vi "Page_Drivers_Write.vi"(6 "ctlReferences":T1, 8 "error in (no error)":errorcluster, 11 "IB_MSI in":refnum<class "IB_MSI.lvclass">) -> (0 "error out":errorcluster, 3 "IB_MSI out":refnum<class "IB_MSI.lvclass">)   [LabVIEW 2020, in "IB_MSI.lvclass"]
uses:
  <vilib>/AppBuilder/IB_Classes/MSI/IB_MSI.lvclass
  <vilib>/AppBuilder/IB_Classes/MSI/IB_MSI.lvclass/IB_MSI.ctl
  <resource>/Framework/Providers/Builds/Installer/Pages/controls/IB_UI_Page_Drivers_References.ctl
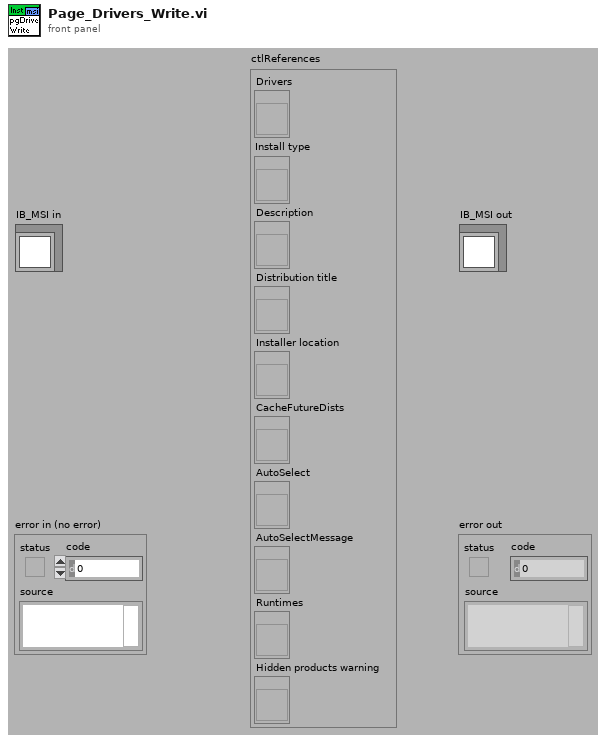
[diagram p1: front panel]
types:
  T1 = typedef "IB_UI_Page_Drivers_References.ctl" = cluster{"Drivers":refnum<vi>, "Install type":refnum<vi>, "Description":refnum<vi>, "Distribution title":refnum<vi>, "Installer location":refnum<vi>, "CacheFutureDists":refnum<vi>, "AutoSelect":refnum<vi>, "AutoSelectMessage":refnum<vi>, "Runtimes":refnum<vi>, "Hidden products warning":refnum<vi>}
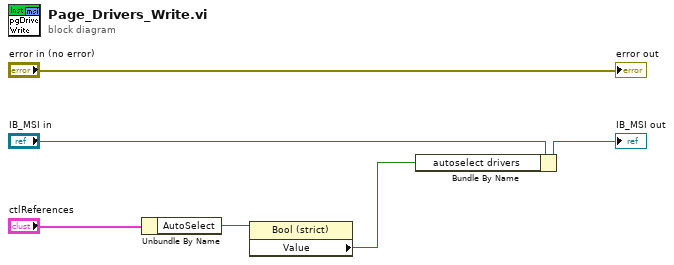
[diagram p0: block diagram]
diagram:
  n1 = Unbundle By Name("ctlReferences") -> ("AutoSelect"=w3:refnum<vi>)
  n2 = property class="Bool (strict)"(reference=w3) -> ("Value"=w2:bool)  [unwired: 1 in, 2 out]
  n3 = Bundle By Name(cluster="IB_MSI in", "autoselect drivers"=w2) -> (→"IB_MSI out":refnum<class "IB_MSI.lvclass">)
  "error out" <- "error in (no error)"
